vi "Write TX.Data.vi"(8 "error in (no error)":errorcluster, 10 "TX.Data":T1 caption="Transmission Data" format="%.0x", 11 "Devices in":refnum<class "Devices.lvclass">) -> (0 "error out":errorcluster, 3 "Devices out":refnum<class "Devices.lvclass">)   [LabVIEW 2020, in "Devices.lvclass"]
uses:
  Devices.lvclass
  TypeDef/Transmission Data.ctl
  Devices.lvclass/Devices.ctl
  I2C Controller Lib.lvlib
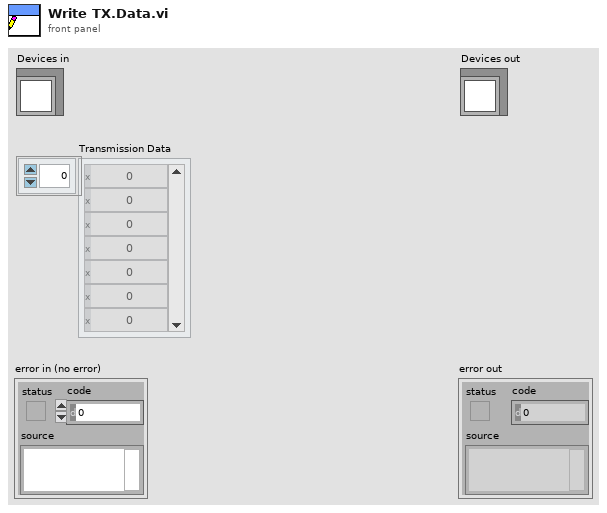
[diagram p1: front panel]
types:
  T1 = typedef "I2C Controller Lib.lvlib/Transmission Data.ctl" = u8[]
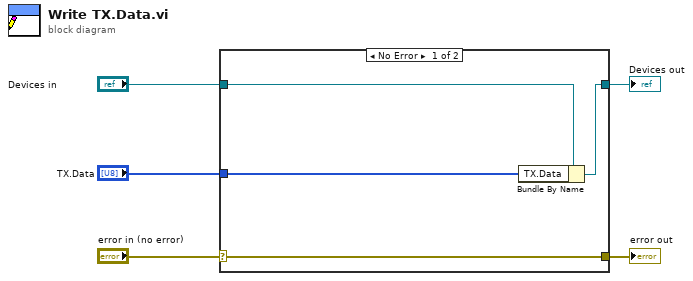
[diagram p0: block diagram]
diagram:
  n1 = case shown="No Error" "error in (no error)" {
    selector: "error in (no error)" -> [w9 w10]
    tunnel: [w9 w10] -> w4
    tunnel: [w7 w11] -> w2
    tunnel: "Devices in" -> [w8 w11]
    tunnel: "TX.Data" -> [w6 _]
    frame No Error {
      n2 = Bundle By Name(cluster=w8, "TX.Data"=w6) -> (w7:refnum<class "Devices.lvclass">)
    }
    frame Error {
    }
  }
  "error out" <- w4
  "Devices out" <- w2
